vi "Display_SetPlayerSelector.vi"(1 "Red in":bool, 2 "Green in":bool, 3 "Blue in":bool, 4 "ActivePixel":T1, 8 "Toggle?":bool) -> (15 "Red out":bool, 16 "Green out":bool, 17 "Blue out":bool, 18 "SelectedNrOfPlayers":T2)   [LabVIEW 2018]
uses:
  TypDefs/Player_Enum.ctl
  TypDefs/ActivePixel_Cluster.ctl
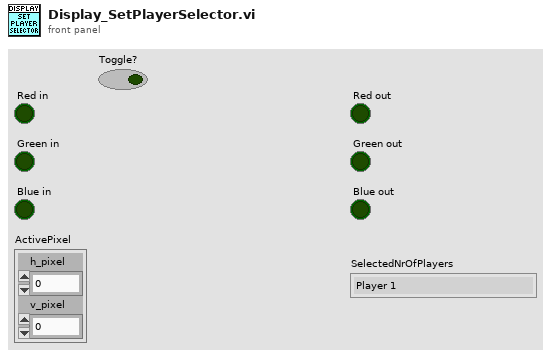
[diagram p1: front panel]
types:
  T1 = typedef "ActivePixel_Cluster.ctl" = cluster{"h_pixel":i16, "v_pixel":i16}
  T2 = typedef "Player_Enum.ctl" = enum16{"Player 1", "Player 2"}
  T3 = cluster{"left":i16, "top":i16, "right":i16, "bottom":i16}
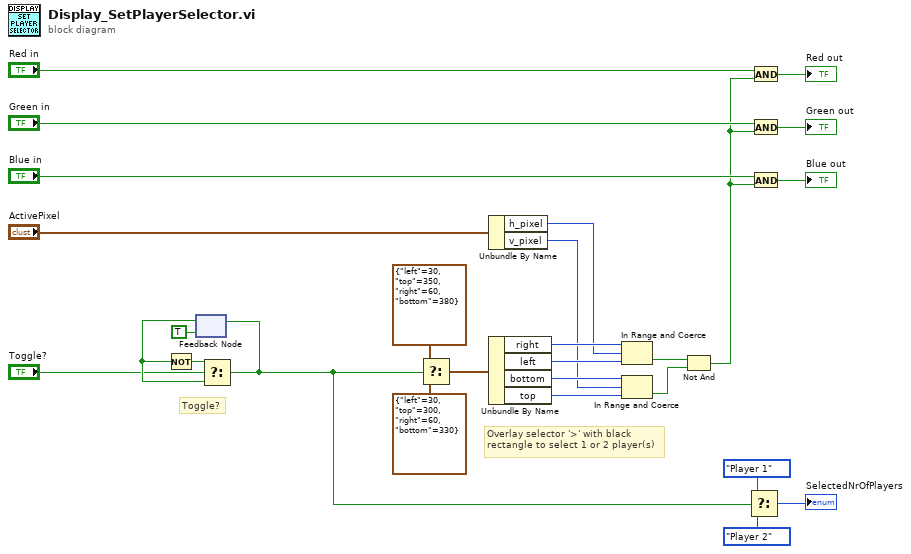
[diagram p0: block diagram]
diagram:
  # "Overlay selector '>' with black\nrectangle to select 1 or 2 player(s)"
  # "Toggle?"
  n1 = feedback #1(TRUE) -> (w3:bool)
  n2 = Not(x=w3) -> (.not. x?=w21:bool)
  n3 = Select(t=w21, s="Toggle?", f=w3) -> (s? t:f=w5:bool)
  n4 = feedback-in #1(w5) -> ()
  n5 = Select(t=T3 {"left"=30, "top"=350, "right"=60, "bottom"=380} ("position"), s=w5, f=T3 {"left"=30, "top"=300, "right"=60, "bottom"=330} ("position")) -> (s? t:f=w20:T3)
  n6 = Unbundle By Name("ActivePixel") -> ("h_pixel"=w10:i16, "v_pixel"=w9:i16)
  n7 = Unbundle By Name(w20) -> ("right"=w22:i16, "left"=w23:i16, "bottom"=w24:i16, "top"=w25:i16)
  n8 = In Range and Coerce(upper limit=w22, x=w10, lower limit=w23) -> (In Range?=w26:bool)  [unwired: 1 out]
  n9 = In Range and Coerce(upper limit=w24, x=w9, lower limit=w25) -> (In Range?=w27:bool)  [unwired: 1 out]
  n10 = Not And(1:w27, 2:w26) -> (0:w4:bool)
  n11 = Select(t=Player_Enum."Player 1" ("Player"), s=w5, f=Player_Enum."Player 2") -> (s? t:f=→"SelectedNrOfPlayers":T2)
  n12 = And(x="Red in", y=w4) -> (x .and. y?=→"Red out":bool)
  n13 = And(x="Green in", y=w4) -> (x .and. y?=→"Green out":bool)
  n14 = And(x="Blue in", y=w4) -> (x .and. y?=→"Blue out":bool)
